vi "element_editor_list_hydrolysis.vi"(10 "Allow all?":bool, 11 "path":path) -> (0 "path to folder":path, 1 "indexes":string[](array[string]), 2 "full_names":string[](array[string]), 3 "Value":string)   [LabVIEW 2019]
panel:
  in  "Button":bool
  in  "Reactors":string(combo)
  # "Choose the reactor:"
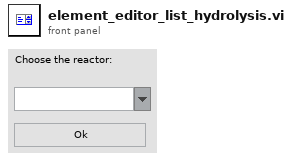
[diagram p1: front panel]
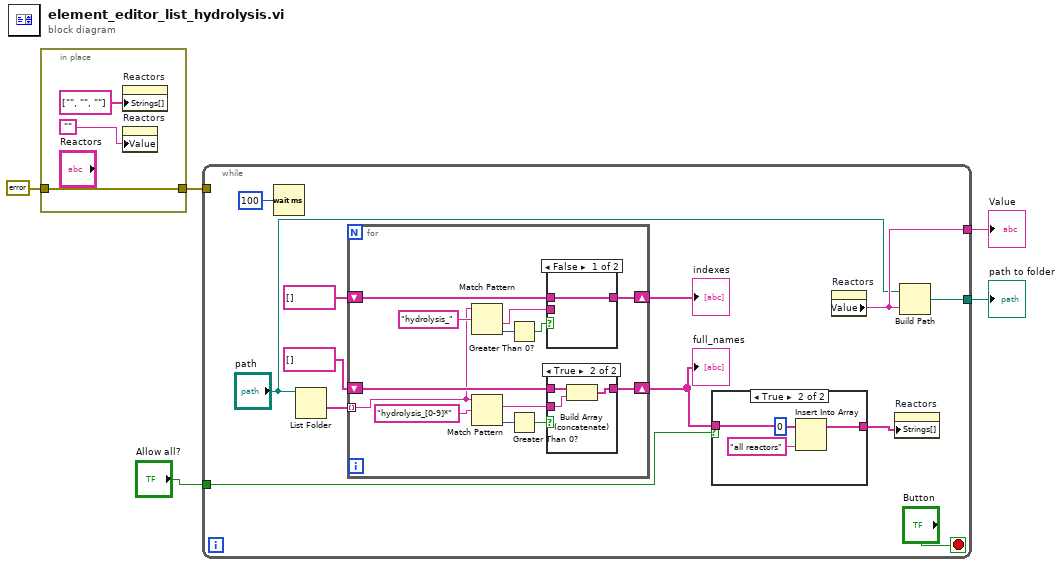
[diagram p0: block diagram]
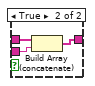
[diagram p3: hidden frame]
diagram:
  n1 = in-place {
    in-place-border: errorcluster {"status"=FALSE, "code"=0, "source"=""} ("error constant") -> [w7]
    in-place-border: [w7] -> w2
    n2 = property on="Reactors" class="CmbBox"("Strings[]"=string[] ["", "", ""] ("full_names")) -> ()  [unwired: 2 in, 2 out]
    n3 = property on="Reactors" class="CmbBox"("Value"="") -> ()  [unwired: 2 in, 2 out]
  }
  n4 = while {
    tunnel: [w14] -> w5
    tunnel: [w12] -> w4
    tunnel: w2 -> [_]
    tunnel: "Allow all?" -> [w9]
    stop <- "Button" stop-if-true
    n5 = Wait (ms)(milliseconds to wait=u32 100) -> ()  [unwired: 1 out]
    n6 = List Folder(path="path") -> (folder names=w20:string[])  [unwired: 3 in, 3 out]
    n7 = for {
      tunnel: w20 -> [w26] mode=indexing
      shift-right: [w33] -> w11
      shift-left: string[] [] -> [w35]
      shift-right: [w29] -> w17
      shift-left: string[] [] ("Array") -> [w28]
      n8 = Match Pattern(string=w26, regular expression="hydrolysis_" ("string")) -> (after substring=w30:string, offset past match=w32:i32)  [unwired: 1 in, 2 out]
      n9 = Match Pattern(string=w26, regular expression="hydrolysis_[0-9]*") -> (match substring=w34:string, offset past match=w36:i32)  [unwired: 1 in, 2 out]
      n10 = Greater Than 0?(x=w32) -> (x > 0?=w31:bool)
      n11 = Greater Than 0?(x=w36) -> (x > 0?=w37:bool)
      n12 = case shown="False" w31 {
        tunnel: w30 -> [_ w42]
        tunnel: [w39 w41] -> w29
        tunnel: w28 -> [w39 w40]
        frame False {
        }
        frame True {
          n13 = Build Array (concatenate)(w40, w42) -> (w41:string[])
        }
      }
      n14 = case shown="True" w37 {
        tunnel: [w43 w46] -> w33
        tunnel: w35 -> [w43 w45]
        tunnel: w34 -> [_ w44]
        frame False {
        }
        frame True {
          n15 = Build Array (concatenate)(w45, w44) -> (w46:string[])
        }
      }
    }
    "full_names" <- w11
    "indexes" <- w17
    n16 = case shown="True" w9 {
      tunnel: w11 -> [w21 w25]
      tunnel: [w21 w24] -> w10
      frame False {
      }
      frame True {
        n17 = Insert Into Array(array=w25, index=0, new element="all reactors" ("new element/subarray")) -> (w24:string[])
      }
    }
    n18 = property on="Reactors" class="CmbBox"() -> ("Value"=w14:string)  [unwired: 2 in, 2 out]
    n19 = property on="Reactors" class="CmbBox"("Strings[]"=w10) -> ()  [unwired: 2 in, 2 out]
    n20 = Build Path(base path="path", name or relative path=w14) -> (appended path=w12:path)
  }
  "Value" <- w5
  "path to folder" <- w4
